vi "SPRACHE.vi"() -> ()   [LabVIEW 2020, in "allgemeine Sub-VIs.lvlib"]
uses:
  allgemeine Sub-VIs.lvlib
  Sprachauswahl native.ctl
  Visualisierungs Elemente/Button.ctl
  Seiten/System Einstellungen V2/Aktioen FGV System Konstanten.ctl
  Seiten/System Einstellungen V2/System Einstellungen V2.lvlib
  Sprachverwaltung/Sprachverwaltung.lvlib
panel:
  in  "Cancel":T1 caption="Abbrechen"
  in  "OK":T1
  in  "Sprache":T2 caption="Bitte wählen Sie eine Sprache:"
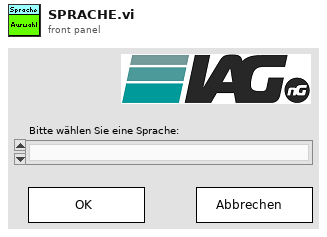
[diagram p1: front panel]
types:
  T1 = typedef "Button.ctl" = bool
  T2 = typedef "Sprachverwaltung.lvlib/Sprachauswahl native.ctl" = u16
  T3 = typedef "System Einstellungen V2.lvlib/Aktioen FGV System Konstanten.ctl" = enum16{"lesen", "laden", "speichern", "Sprache"}
  T4 = typedef "LVStringsAndValuesArrayTypeDef_U16.ctl" = cluster{"String":string, "Value":u16}[]
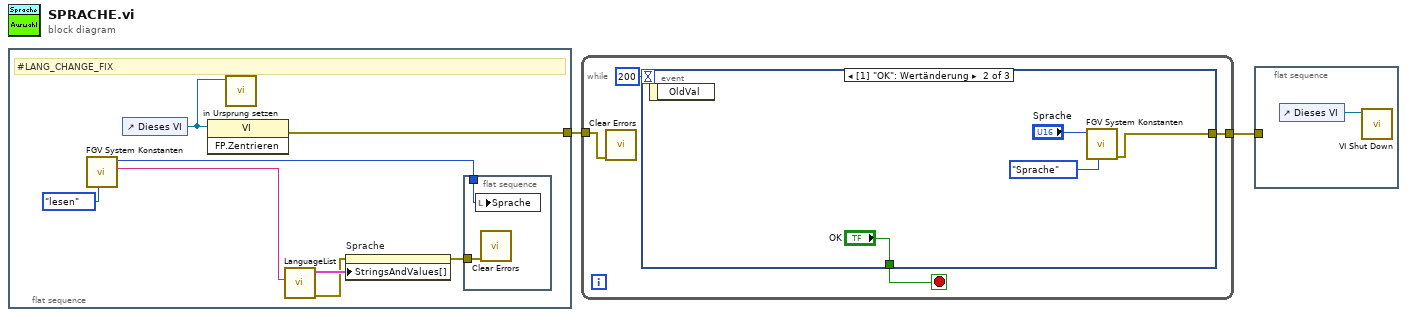
[diagram p0: block diagram]
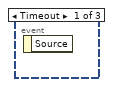
[diagram p2: hidden frame]
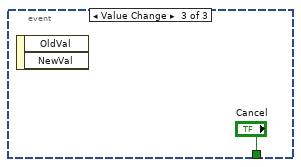
[diagram p3: hidden frame]
diagram:
  n1 = flat-sequence {
    tunnel: [w9] -> w2
    frame #0 {
      # "#LANG_CHANGE_FIX"
      n2 = call "FGV System Konstanten.vi"("Aktionen"=Aktioen_FGV_System_Konstanten."lesen") -> ("LanguageList"=w3:string, "Sprachindex"=w6:u16)  [unwired: 6 in, 3 out]
      n3 = control-ref of="Dieses VI"() -> (w10:refnum<vi>)
      n4 = invoke class="VI" method="FP.Zentrieren"(reference=w10) -> (error out=w9:errorcluster)  [unwired: 2 in, 2 out]
      n5 = call "in Ursprung setzen.vi"("VI Referenz"=w10) -> ()  [unwired: 10 in, 1 out]
      n6 = call "LanguageList.vi"("LanguageList"=w3) -> ("Fehler (Ausgang)"=w4:errorcluster, "Strings und Werte []"=w8:T4)  [unwired: 5 in, 4 out]
      n7 = property on="Sprache" class="Ring (strikt)"(error in=w4, "StringsAndValues[]"=w8) -> (error out=w7:errorcluster)  [unwired: 1 in, 1 out]
      n8 = flat-sequence {
        tunnel: w6 -> [w11]
        tunnel: w7 -> [w12]
        frame #0 {
          n9 = local write "Sprache"(w11) -> ()
          n10 = call <vilib>:"Clear Errors.vi"("error in (no error)"=w12) -> ()  [unwired: 5 in, 2 out]
        }
      }
    }
  }
  n11 = while {
    tunnel: w2 -> [w14]
    tunnel: [w13] -> w1
    stop <- w15 stop-if-true
    n12 = call <vilib>:"Clear Errors.vi"("error in (no error)"=w14) -> ()  [unwired: 5 in, 2 out]
    n13 = event shown="[1] \"OK\": Wertänderung" {
      selector: _ -> [_ _ _]
      dyn-events: _ -> [_ _ _]
      timeout: 200 -> [_ _ _]
      tunnel: [_ "OK" "Cancel"] -> w15
      tunnel: [_ w17 _] -> w13
      event Timeout {
        n14 = event-data() -> ()  [unwired: 1 in, 1 out]
      }
      event Value Change {
        n15 = event-data() -> ()  [unwired: 1 in, 1 out]
        n16 = call "FGV System Konstanten.vi"("Aktionen"=Aktioen_FGV_System_Konstanten."Sprache", "Sprache"="Sprache") -> ("error out"=w17:errorcluster)  [unwired: 5 in, 4 out]
      }
      event Value Change {
        n17 = event-data() -> ()  [unwired: 1 in, 2 out]
      }
    }
  }
  n18 = flat-sequence {
    tunnel: w1 -> [_]
    frame #0 {
      n19 = control-ref of="Dieses VI"() -> (w22:refnum<vi>)
      n20 = call "VI Shut Down.vi"("VI Referenz"=w22) -> ()  [unwired: 11 in]
    }
  }
